vi "Create Concrete Message for Method.vi"(6 "Project Path":path, 8 "error in (no error)":errorcluster, 9 "Item Refnum":refnum<vi>, 10 "Target":refnum<vi>) -> (0 "error out":errorcluster)   [LabVIEW 2020, in "Message Maker Provider.lvlib"]
uses:
  Message Maker Provider.lvlib
  _Message Maker/_Maker Classes/Message Scripter/Message Scripter.lvclass
  _Message Maker/_Maker Classes/Concrete Message Scripter/Concrete Message Scripter.lvclass
  _Message Maker/_Maker Classes/Target Method Icon Reader/Target Method Icon Reader.lvclass
  Localized Strings.vi
panel:
  out "New Send Method":path
  out "New Class Path":path
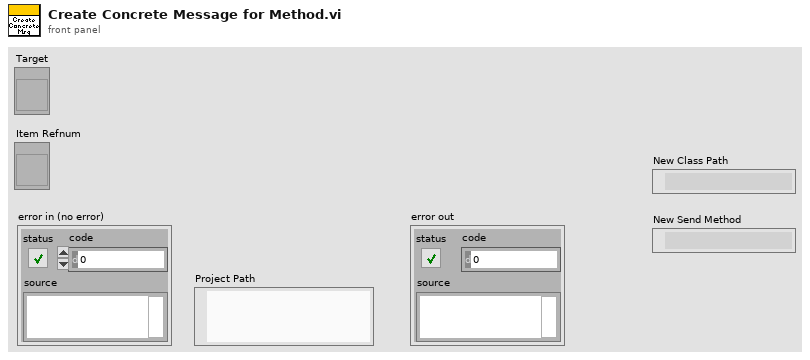
[diagram p1: front panel]
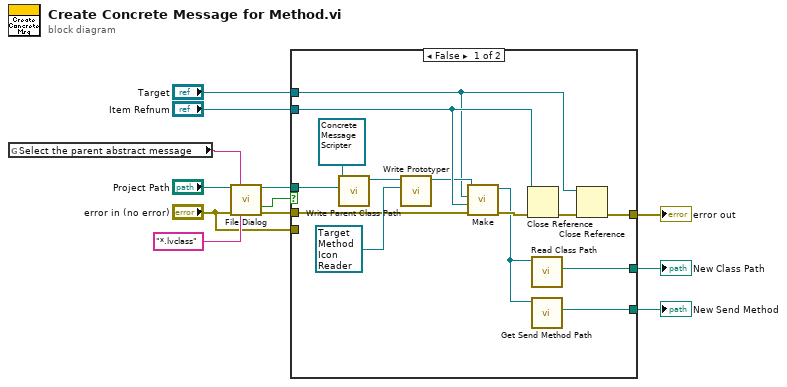
[diagram p0: block diagram]
diagram:
  n1 = global read "Localized Strings.vi" "Select the parent abstract message"() -> (w1:string)
  n2 = call "File Dialog"("start path"="Project Path", "prompt"=w1, "error in"="error in (no error)", "pattern (all files)"="*.lvclass") -> ("selected path"=w9:path, "cancelled"=w10:bool, "error out"=w11:errorcluster)  [unwired: 8 in, 1 out]
  n3 = case shown="False" w10 {
    tunnel: [w25 w27] -> w2
    tunnel: w11 -> [w14 _]
    tunnel: w9 -> [w23 _]
    tunnel: "Target" -> [w13 _]
    tunnel: "Item Refnum" -> [w24 _]
    tunnel: [w20 _] -> w5
    tunnel: [w19 _] -> w4
    tunnel: "error in (no error)" -> [_ w27]
    frame False {
      n4 = call-dynamic "Write Parent Class Path.vi"("Parent Class Path"=w23, "Concrete Message Scripter in"=refnum<class "Concrete Message Scripter.lvclass"> refnum ("Message Maker.lvlib:Concrete Message Scripter.lvclass")) -> ("Concrete Message Scripter out"=w17:refnum<class "Concrete Message Scripter.lvclass">)  [unwired: 9 in]
      n5 = call "Write Prototyper.vi"("Prototyper"=refnum<class "Target Method Icon Reader.lvclass"> refnum ("Message Maker.lvlib:Target Method Icon Reader.lvclass"), "Message Scripter in"=w17) -> ("Message Scripter out"=w16:refnum<class "Concrete Message Scripter.lvclass">)  [unwired: 9 in]
      n6 = call-dynamic "Make.vi"("error in (no error)"=w14, "Item Refnum"=w24, "Target"=w13, "Concrete Message Scripter"=w16) -> ("error out"=w22:errorcluster, "Concrete Message Scripter out"=w21:refnum<class "Concrete Message Scripter.lvclass">)  [unwired: 6 in]
      n7 = Close Reference(reference=w24, error in (no error)=w22) -> (error out=w26:errorcluster)
      n8 = call "Read Class Path.vi"("Message Scripter in"=w21) -> ("Class Path"=w20:path)  [unwired: 10 in]
      n9 = call "Get Send Method Path.vi"("Message Scripter"=w21) -> ("Send Method Path"=w19:path)  [unwired: 10 in]
      n10 = Close Reference(reference=w13, error in (no error)=w26) -> (error out=w25:errorcluster)
    }
    frame True {
    }
  }
  "error out" <- w2
  "New Class Path" <- w5
  "New Send Method" <- w4
